vi "Config_Image_Read_DetectorROIs.vi"(8 "error in (no error)":errorcluster) -> (0 "error out":errorcluster)   [LabVIEW 2020]
uses:
  <vilib>/Utility/config.llb/Read Key (String).vi
  <vilib>/Utility/config.llb/NI_LVConfig.lvlib
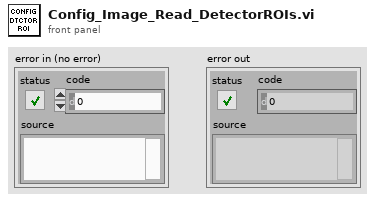
[diagram p1: front panel]
types:
  T1 = typedef "Image_Cluster.ctl" = cluster{"Detector_info":cluster{"No. of detectors":dbl, "Detector_Array":string[][], "Detector_Array_Numeric":dbl[][]}, "Corner_info":cluster{"Corner_Array":dbl[][]}, "ROI":cluster{"Corners":cluster{"Global Rectangle":i32[], "Contours":cluster{"ID":enum32{"External", "Internal"}, "Type":u32, "Coordinates":i32[]}[]}[], "Detectors":cluster{"Global Rectangle":i32[], "Contours":cluster{"ID":enum32{"External", "Internal"}, "Type":u32, "Coordinates":i32[]}[]}[]}, "Shape_Detect":cluster{"Match_score":dbl, "Curve Parameters":T2, "Match Options":T3, "Circle Descriptor":cluster{"Min Radius":dbl, "Max Radius":dbl}}, "Path":cluster{"Config":path, "Map":path}, "Map":cluster{"X_resolution":i32, "Y_resolution":i32, "Image":T5, "Image_colored":T5}, "Conversion_factor":dbl}
  T2 = typedef "IMAQ Curve Parameters.ctl" = cluster{"Extraction Mode":u32, "Edge Threshold":i32, "Edge Filter Size":u32, "Min Length":i32, "Row Search Step Size":i32, "Col Search Step Size":i32, "Max Endpoint Gap":i32, "Closed":bool, "Subpixel":bool}
  T3 = typedef "ShapeDetectionMatchOptions.ctl" = cluster{"Rotation":bool, "Scale":bool, "Occlusion":bool, "Range Settings":T4[]}
  T4 = typedef "IMAQ Match Range Setting.ctl" = cluster{"Match Constraints":u32, "Min":dbl, "Max":dbl}
  T5 = typedef "IMAQ Image.ctl" = refnum<image>
  T6 = typedef "NI_LVConfig.lvlib/Config Data RefNum.ctl" = refnum<k1>
  T7 = cluster{"Global Rectangle":i32[], "Contours":cluster{"ID":enum32{"External", "Internal"}, "Type":u32, "Coordinates":i32[]}[]}
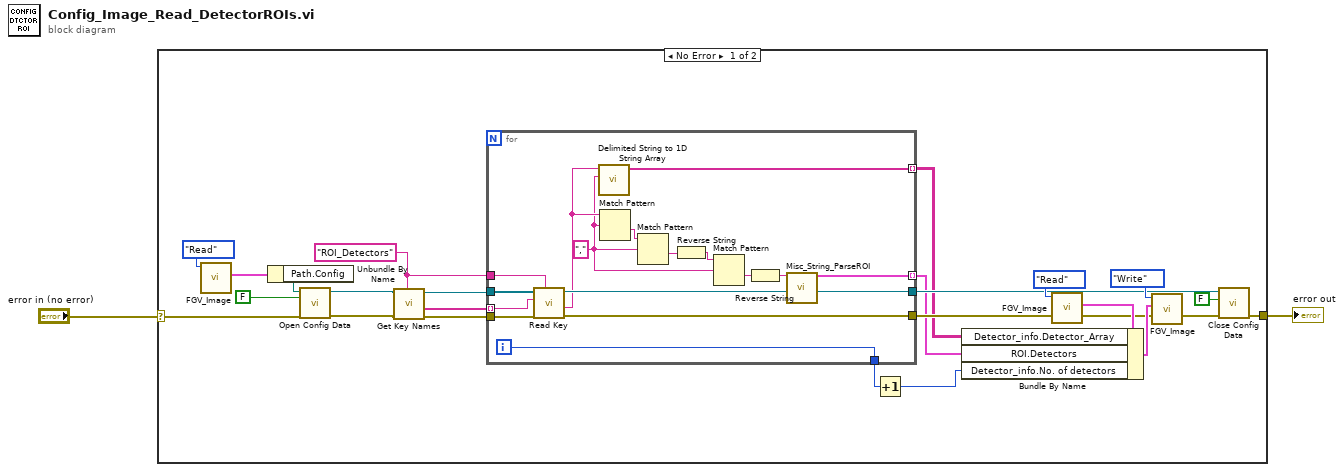
[diagram p0: block diagram]
diagram:
  n1 = case shown="No Error" "error in (no error)" {
    selector: "error in (no error)" -> [w15 w42]
    tunnel: [w25 w42] -> w2
    frame No Error {
      w9 = "ROI_Detectors"
      n2 = call "FGV_Image.vi"("Action"=enum16{"Read", "Write", ""}."Read") -> ("Image_Cluster_out"=w23:T1)  [unwired: 10 in]
      n3 = Unbundle By Name(w23) -> ("Path.Config"=w24:path)
      n4 = call <vilib>:"Open Config Data.vi"("error in (no error)"=w15, "create file if necessary (T)"=FALSE, "configuration file path"=w24) -> ("error out"=w14:errorcluster, "refnum"=w13:T6)  [unwired: 6 in, 1 out]
      n5 = call <vilib>:"Get Key Names.vi"("section"=w9, "error in (no error)"=w14, "refnum"=w13) -> ("error out"=w11:errorcluster, "key names"=w12:string[], "refnum out"=w8:T6)  [unwired: 5 in, 1 out]
      n6 = for {
        tunnel: w12 -> [w39] mode=indexing
        tunnel: w11 -> [w41]
        tunnel: [w40] -> w10
        tunnel: w9 -> [w38]
        tunnel: w8 -> [w37]
        tunnel: [w36] -> w7
        tunnel: [w30] -> w6 mode=indexing
        tunnel: [w27] -> w5 mode=indexing
        tunnel: [w26] -> w3
        i -> [w26]
        w28 = "," ("regular expression")
        n7 = call-poly <vilib>:"Read Key.vi"("section"=w38, "error in (no error)"=w41, "key"=w39, "refnum"=w37) -> ("error out"=w40:errorcluster, "value"=w29:string, "refnum out"=w36:T6)  [unwired: 4 in, 1 out]
        n8 = call <vilib>:"Delimited String to 1D String Array.vi"("delimiter"=w28, "delimited string"=w29) -> ("string array"=w27:string[])  [unwired: 9 in]
        n9 = Match Pattern(string=w29, regular expression=w28) -> (after substring=w35:string)  [unwired: 1 in, 3 out]
        n10 = Match Pattern(string=w35, regular expression=w28) -> (after substring=w34:string)  [unwired: 1 in, 3 out]
        n11 = Reverse String(1:w34) -> (0:w33:string)
        n12 = Match Pattern(string=w33, regular expression=w28) -> (after substring=w32:string)  [unwired: 1 in, 3 out]
        n13 = Reverse String(1:w32) -> (0:w31:string)
        n14 = call "Misc_String_ParseROI.vi"("ROI_string"=w31) -> ("ROI"=w30:T7)  [unwired: 14 in]
      }
      n15 = Increment(x=w3) -> (x+1=w4:i32)
      n16 = call "FGV_Image.vi"("Action"=enum16{"Read", "Write", ""}."Read") -> ("Image_Cluster_out"=w19:T1)  [unwired: 10 in]
      n17 = Bundle By Name(cluster=w19, "Detector_info.Detector_Array"=w5, "ROI.Detectors"=w6, "Detector_info.No. of detectors"=w4) -> (w20:T1)
      n18 = call "FGV_Image.vi"("Image_Cluster_in"=w20, "Action"=enum16{"Read", "Write", ""}."Write") -> ()  [unwired: 9 in, 1 out]
      n19 = call <vilib>:"Close Config Data.vi"("error in (no error)"=w10, "write file if changed (T)"=FALSE ("write configuration file? (T)"), "refnum"=w7) -> ("error out"=w25:errorcluster)  [unwired: 8 out]
    }
    frame Error {
    }
  }
  "error out" <- w2
